vi "demo_ee2.vi"() -> ()   [LabVIEW 2018]
doc: "演示设置基本TCP连接、建立连接后发送数据至指定端口并在完成发送后中止连接的方法。VI设计为TCP连接断开时停止。本范例中发送的数据为随机数数组。"
uses:
  <vilib>/addons/control/pid/NI_PID_autopid.lvlib
panel:
  out "力初始位移":dbl
  out "前馈输出":dbl
  in  "Lower Cut-Off 2":dbl=5.0 caption="截止频率2"
  in  "Lower Cut-Off 1":dbl=5.0 caption="截止频率1"
  out "PID输出":dbl
  in  "重力补偿":dbl=1.15
  in  "力控制频率":dbl=100.0
  in  "位移模块":path caption="文件名"
  in  "力模块":path caption="文件名"
  in  "stop (F) 2":bool caption="停止力控"
  out "力控模块\n气压-位移-力":dynamicdata(graph)
  in  "PID gains":T1={"proportional gain (Kc)"=0.25, "integral time (Ti, min)"=0.05, "derivative time (Td, min)"=0.0} caption="PID增益" {"derivative time (Td, min)" format="%.3f"; "integral time (Ti, min)" format="%.3f"; "proportional gain (Kc)" format="%.3f"}
  in  "output range":cluster{"output high":dbl, "output low":dbl}={"output high"=0.2, "output low"=-0.2} caption="输出范围" {"output low" format="%.2f"; "output high" format="%.2f"}
  in  "a 斜率":dbl=-0.33869
  in  "b 截距":dbl=10.683
  in  "设定力Fd/N":dbl=10.0
  out "力 /N":dynamicdata(graph)
  out "力控模块指令":string
  out "力初始气压":dbl
  in  "stop (F)":bool caption="停止\n位控"
  out "位移模块\n气压-位移-力":dynamicdata(graph)
  in  "位置控制频率":dbl=100.0
  in  "移动速率 mm/s":dbl=0.5
  in  "Flag":i8=2
  out "1/u":dbl(graph)
  in  "力阈值F0/N":dbl=2.0
  out "位置初始气压":dbl
  in  "停止气压":dbl(slide)=4.5 scale=2.5..5.0
  in  "停止 2":bool
  in  "初始气压 /bar":dbl=4.5
  in  "停止":bool
  out "位置模块指令":string
  # "FLag: 1 上升\n        2 下降"
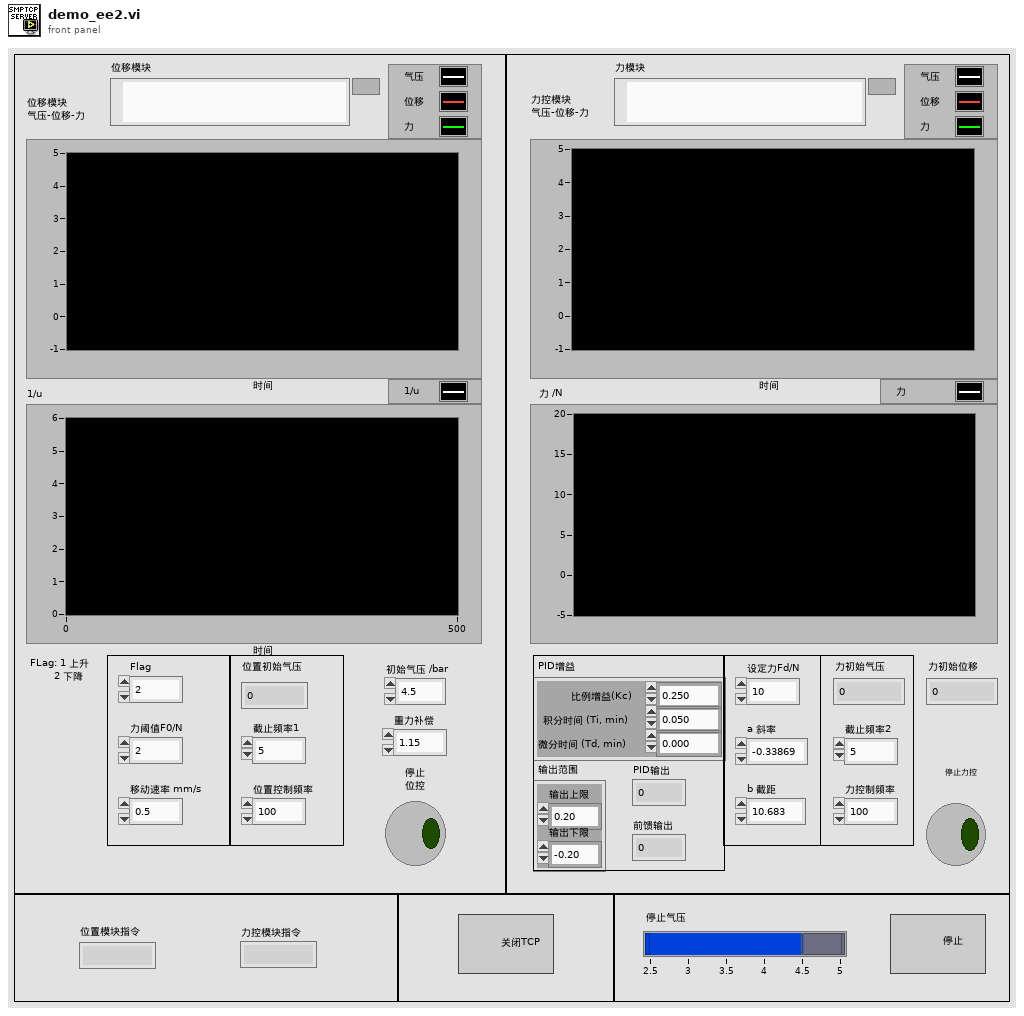
[diagram p1: front panel]
types:
  T1 = cluster{"proportional gain (Kc)":dbl, "integral time (Ti, min)":dbl, "derivative time (Td, min)":dbl}
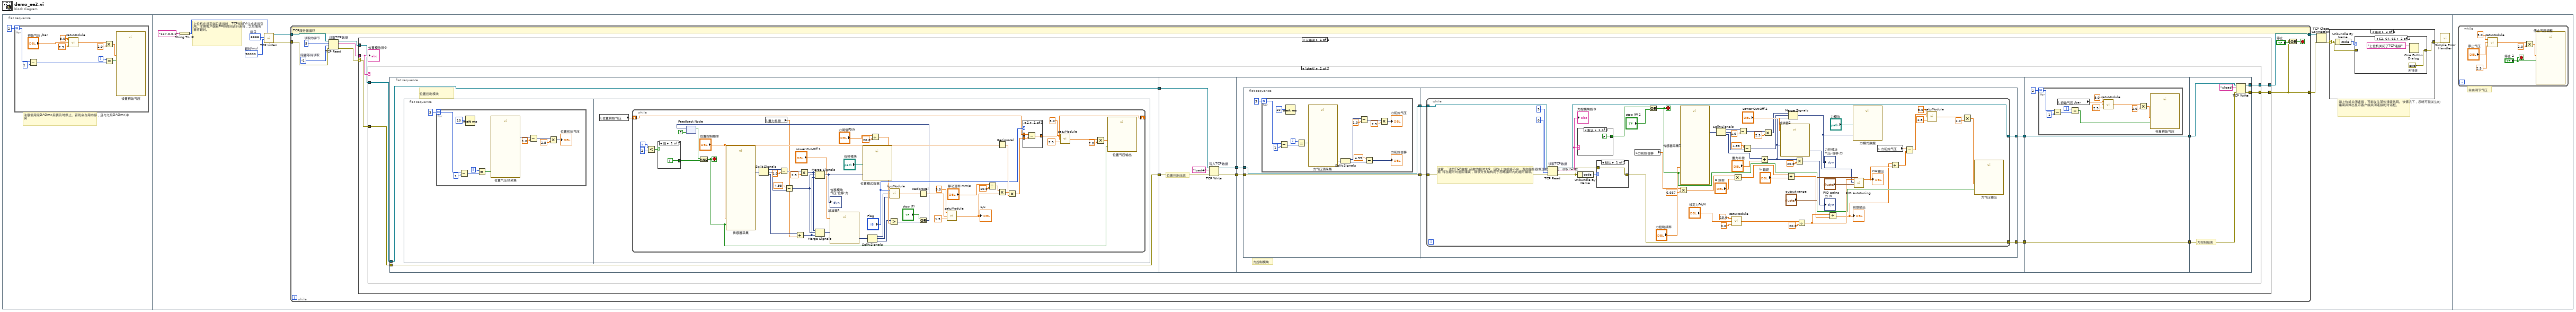
[diagram p0: block diagram]
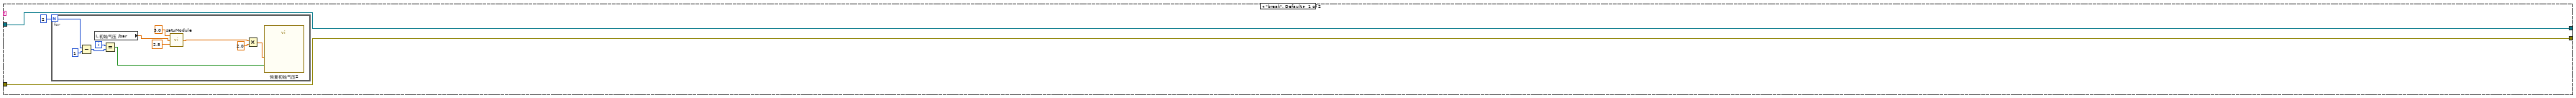
[diagram p4: hidden frame]
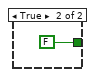
[diagram p5: hidden frame]
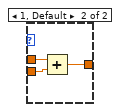
[diagram p6: hidden frame]
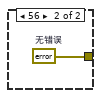
[diagram p7: hidden frame]
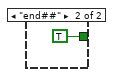
[diagram p8: hidden frame]
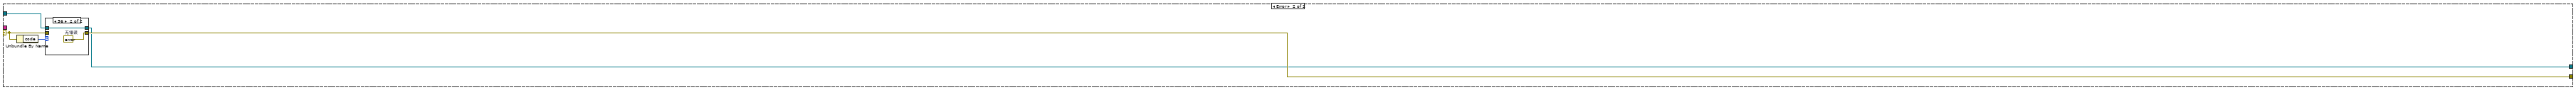
[diagram p9: hidden frame]
diagram:
  n1 = flat-sequence {
    frame #0 {
      # "注意使用完DAQmx后要及时停止。否则会占用内存，且与之后DAQmx冲突"
      n2 = for {
        N: 2 -> [w4]
        i -> [w6]
        n3 = Subtract(x=w4, y=1) -> (x-y=w2:i32)
        n4 = call "satuModule.vi"("min"=2.5, "input"="初始气压 /bar", "max"=5.0) -> ("output"=w11:dbl)
        n5 = Multiply(x=w11, y=2.0 ("x")) -> (x*y=w12:dbl)
        n6 = Equal?(x=w6, y=w2) -> (x = y?=w5:bool)
        n7 = call "设置初始气压"("data"=w12, "stop (T)"=w5) -> ()  [unwired: 16 in, 2 out]
      }
    }
    frame #1 {
      w19 = u16 6666  # 端口
      w20 = 90000  # 超时(ms)
      # "如上位机关闭连接，可能发生某些错误代码。该情况下，忽略可能发生的错误并弹出显示客户端关闭连接的对话框。"
      # "上位机在指定端口连接时，TCP侦听VI生成连接引用。注意客户端有90秒时间进行连接，之后服务器将超时。"
      n8 = String To IP(1:"127.0.0.1") -> (0:w18:u32)
      n9 = call <vilib>:"TCP Listen.vi"("net address"=w18, "timeout ms (wait forever: -1)"=w20, "port"=w19) -> ("error out"=w21:errorcluster, "connection ID"=w22:refnum<k5>)  [unwired: 4 in, 3 out]
      n10 = while {
        tunnel: [w38] -> w13
        tunnel: w22 -> [w37]
        tunnel: w21 -> [w36]
        tunnel: [w32] -> w14
        stop <- w40 stop-if-true
        w30 = -1  # 阻塞等待读取
        w35 = 5  # 读取的字节
        # "TCP服务器循环"
        n11 = TCP Read "读取TCP数据"(connection ID=w37, bytes to read=w35, error in (no error)=w36, 9:w30) -> (connection ID out=w33:refnum<k5>, data out=w31:string, error out=w34:errorcluster)  [unwired: 1 in]
        n12 = case shown="无错误" w34 {
          selector: w34 -> [w43 w263]
          tunnel: [w42 w262] -> w38
          tunnel: w33 -> [w44 w261]
          tunnel: [w41 w260] -> w32
          tunnel: w31 -> [w45 _]
          frame No Error {
            n13 = case shown="\"start\"" w45 {
              tunnel: w44 -> [w47 w64]
              tunnel: w43 -> [w48 w71]
              tunnel: [w48 w69] -> w42
              tunnel: [w47 w66] -> w41
              frame "break", Default {
                n14 = for {
                  N: 2 -> [w53]
                  i -> [w50]
                  n15 = Subtract(x=w53, y=1) -> (x-y=w51:i32)
                  n16 = local read "初始气压 /bar"() -> (w54:dbl)
                  n17 = Equal?(x=w50, y=w51) -> (x = y?=w49:bool)
                  n18 = call "satuModule.vi"("min"=2.5, "input"=w54, "max"=5.0) -> ("output"=w58:dbl)
                  n19 = Multiply(x=w58, y=2.0 ("x")) -> (x*y=w59:dbl)
                  n20 = call "恢复初始气压2"("data"=w59, "stop (T)"=w49) -> ()  [unwired: 16 in, 2 out]
                }
              }
              frame "start" {
                n21 = flat-sequence {
                  tunnel: w71 -> [w73]
                  tunnel: [w73] -> w70
                  tunnel: [w72] -> w65
                  tunnel: w64 -> [w72]
                  tunnel: w70 -> [w151]
                  tunnel: [w150] -> w68
                  tunnel: [w149] -> w67
                  tunnel: w65 -> [w148]
                  tunnel: w68 -> [w155]
                  tunnel: w67 -> [w157]
                  tunnel: [w154] -> w62
                  tunnel: [w153] -> w60
                  tunnel: [w243] -> w63
                  tunnel: w62 -> [w243]
                  tunnel: [w242] -> w61
                  tunnel: w60 -> [w242]
                  tunnel: [w258] -> w66
                  tunnel: [w257] -> w69
                  tunnel: w63 -> [w256]
                  tunnel: w61 -> [w255]
                  frame #0 {
                    # "位置控制模块"
                    n22 = flat-sequence {
                      frame #0 {
                        n23 = for {
                          N: 3 -> [w77]
                          i -> [w80]
                          n24 = Subtract(x=w77, y=1) -> (x-y=w75:i32)
                          n25 = Wait (ms)(milliseconds to wait=u32 10 ("等待时间（毫秒）")) -> ()  [unwired: 1 out]
                          n26 = Equal?(x=w80, y=w75) -> (x = y?=w79:bool)
                          n27 = call "位置气压预采集"("stop (T)"=w79) -> ("data"=w82:dynamicdata)  [unwired: 16 in, 2 out]
                          n28 = Subtract(x=w82, y=1.0) -> (x-y=w85:dynamicdata)
                          n29 = Multiply(x=w85, y=2.5) -> (x*y=→"位置初始气压":dynamicdata)
                        }
                      }
                      frame #1 {
                        n30 = local read "位置初始气压"() -> (w86:dbl)
                        n31 = while {
                          shift-right: [w113] -> _
                          shift-left: w86 -> [w112]
                          i -> [w100]
                          stop <- w101 stop-if-true
                          n32 = Less?(x=w100, y=2) -> (x < y?=w98:bool)
                          n33 = case shown="假" w98 {
                            tunnel: [TRUE FALSE] -> w97
                            frame False {
                            }
                            frame True {
                            }
                          }
                          n34 = feedback #1(FALSE) -> (w102:bool)
                          n35 = And(x=w102, y=w97) -> (x .and. y?=w101:bool)
                          n36 = call "传感器采集"("速率"="位置控制频率", "stop (F)"=w101) -> ("data"=w136:dynamicdata)  [unwired: 14 in, 3 out]
                          n37 = Split Signals(w136) -> (w135:dynamicdata, w133:dynamicdata, w130:dynamicdata)  [unwired: 3 in]
                          n38 = local read "重力补偿"() -> (w96:dbl)
                          n39 = Subtract(x=w135, y=1.0) -> (x-y=w138:dynamicdata)
                          n40 = Subtract(x=4.95, y=w133) -> (x-y=w94:dynamicdata)
                          n41 = Add(x=w130, y=w96) -> (x+y=w93:dynamicdata)
                          n42 = Multiply(x=w138, y=2.5) -> (x*y=w95:dynamicdata)
                          n43 = Merge Signals(w95, w94, w93) -> (w107:dynamicdata)
                          "位移模块\n气压-位移-力" <- w107
                          n44 = Merge Signals(w95, w94, w93) -> (w92:dynamicdata)
                          n45 = call "滤波器1"("Lower Cut-Off"="Lower Cut-Off 1", "Signal"=w92) -> ("Filtered Signal"=w87:dynamicdata)  [unwired: 8 in, 1 out]
                          n46 = call "位置模式数据"("Signals"=w107, "Filename"="位移模块") -> ()  [unwired: 15 in, 3 out]
                          n47 = Split Signals(w87) -> (w91:dynamicdata, w90:dynamicdata, w89:dynamicdata)  [unwired: 3 in]
                          n48 = Divide(x="力阈值F0/N", y=20.0) -> (x/y=w109:dbl)
                          n49 = Greater?(x=w89, y=w109) -> (0:w105:dynamicdata)
                          n50 = call "hysModule.vi"("cur_x"=w90, "cur_p"=w91, "flag"="Flag") -> ("u"=w116:dbl)
                          n51 = Reciprocal(x=w116) -> (1/x=w115:dbl)
                          n52 = Or(x="stop (F)", y=w105) -> (x .or. y?=w104:dynamicdata)
                          n53 = feedback-in #1(w104) -> ()
                          n54 = call "satuModule.vi"("min"=1.5, "input"=w115, "max"=5.0) -> ("output"=w114:dbl)
                          "1/u" <- w114
                          n55 = Divide(x="移动速率 mm/s", y=10.0) -> (x/y=w124:dbl)
                          n56 = Reciprocal(x="位置控制频率") -> (1/x=w121:dbl)
                          n57 = Multiply(x=w124, y=w114) -> (x*y=w122:dbl)
                          n58 = Multiply(x=w122, y=w121) -> (x*y=w119:dbl)
                          n59 = case shown="2" "Flag" {
                            tunnel: [w144 w147] -> w113
                            tunnel: w119 -> [w143 w146]
                            tunnel: w112 -> [w142 w145]
                            frame 2 {
                              n60 = Subtract(x=w142, y=w143) -> (x-y=w144:dbl)
                            }
                            frame 1, Default {
                              n61 = Add(x=w145, y=w146) -> (x+y=w147:dbl)
                            }
                          }
                          n62 = call "satuModule.vi"("min"=2.5, "input"=w113, "max"=5.0) -> ("output"=w127:dbl)
                          n63 = Multiply(x=w127, y=2.0 ("x")) -> (x*y=w132:dbl)
                          n64 = call "位置气压输出"("data"=w132, "stop (T)"=w101) -> ()  [unwired: 16 in, 2 out]
                        }
                      }
                    }
                  }
                  frame #1 {
                    # "位置控制结束"
                    n65 = TCP Write "写入TCP数据"(connection ID=w148, data in="load#" ("数据输入"), error in (no error)=w151) -> (connection ID out=w149:refnum<k5>, error out=w150:errorcluster)  [unwired: 2 out]
                  }
                  frame #2 {
                    # "力控制模块"
                    n66 = flat-sequence {
                      tunnel: [w161] -> w158
                      tunnel: w157 -> [w161]
                      tunnel: [w160] -> w156
                      tunnel: w155 -> [w160]
                      tunnel: w158 -> [w180]
                      tunnel: w156 -> [w179]
                      tunnel: [w178] -> w154
                      tunnel: [w177] -> w153
                      frame #0 {
                        n67 = for {
                          N: 3 -> [w169]
                          i -> [w172]
                          n68 = Subtract(x=w169, y=1) -> (x-y=w168:i32)
                          n69 = Wait (ms)(milliseconds to wait=u32 10 ("等待时间（毫秒）")) -> ()  [unwired: 1 out]
                          n70 = Equal?(x=w172, y=w168) -> (x = y?=w171:bool)
                          n71 = call "力气压预采集"("stop (T)"=w171) -> ("data"=w166:dynamicdata)  [unwired: 16 in, 2 out]
                          n72 = Split Signals(w166) -> (w165:dynamicdata, w164:dynamicdata)  [unwired: 2 in]
                          n73 = Subtract(x=w165, y=1.0) -> (x-y=w176:dynamicdata)
                          n74 = Subtract(x=4.95, y=w164) -> (x-y=→"力初始位移":dynamicdata)
                          n75 = Multiply(x=w176, y=2.5) -> (x*y=→"力初始气压":dynamicdata)
                        }
                      }
                      frame #1 {
                        n76 = while {
                          tunnel: w180 -> [w199]
                          tunnel: w179 -> [w198]
                          tunnel: [w197] -> w178
                          tunnel: [w196] -> w177
                          stop <- w192 stop-if-true
                          # "注意，“读取TCP数据”函数的超时为0，因为上位机将不会一直向服务器发送数据。由于“读取TCP数据”将在超时时返回错误，错误分支结构用于忽略循环内的超时错误。"
                          n77 = TCP Read "读取TCP数据"(connection ID=w199, bytes to read=5 ("读取的字节"), error in (no error)=w198, 9:0 ("超时毫秒(25000)")) -> (connection ID out=w197:refnum<k5>, data out=w204:string, error out=w200:errorcluster)  [unwired: 1 in]
                          "力控模块指令" <- w204
                          n78 = case shown="默认" w204 {
                            tunnel: [FALSE TRUE] -> w202
                            frame Default {
                            }
                            frame "end##" {
                            }
                          }
                          n79 = Unbundle By Name(w200) -> ("code"=w201:i32)
                          n80 = case shown="默认" w201 {
                            tunnel: w200 -> [w237 _]
                            tunnel: [w237 w238] -> w196
                            frame Default {
                            }
                            frame 56 {
                              w238 = errorcluster {"status"=FALSE, "code"=0, "source"=""}  # 无错误
                            }
                          }
                          n81 = local read "力初始位移"() -> (w182:dbl)
                          n82 = Or(x=w202, y="stop (F) 2") -> (x .or. y?=w192:bool)
                          n83 = Multiply(x=w182, y=6.667) -> (x*y=w227:dbl)
                          n84 = call "传感器采集2"("速率"="力控制频率", "stop (F)"=w192) -> ("data"=w233:dynamicdata)  [unwired: 14 in, 3 out]
                          n85 = Split Signals(w233) -> (w223:dynamicdata, w221:dynamicdata, w220:dynamicdata)  [unwired: 3 in]
                          n86 = call "satuModule.vi"("min"=0.0 ("下限"), "input"="设定力Fd/N", "max"=15.0) -> ("output"=w213:dbl)
                          n87 = Multiply(x=w227, y="a 斜率") -> (x*y=w224:dbl)
                          n88 = Subtract(x=w223, y=1.0) -> (x-y=w235:dynamicdata)
                          n89 = Subtract(x=4.95, y=w221) -> (x-y=w186:dynamicdata)
                          n90 = Add(x=w220, y="重力补偿") -> (x+y=w184:dynamicdata)
                          n91 = Multiply(x=w235, y=2.5) -> (x*y=w187:dynamicdata)
                          n92 = call "滤波器2"("Lower Cut-Off"="Lower Cut-Off 2", "Signal"=w184) -> ("Filtered Signal"=w183:dynamicdata)  [unwired: 8 in, 1 out]
                          n93 = Add(x=w224, y="b 截距") -> (x+y=w181:dbl)
                          n94 = Merge Signals(w187, w186, w184) -> (w195:dynamicdata)
                          "力控模块\n气压-位移-力" <- w195
                          n95 = Multiply(x=w184, y=20.0) -> (x*y=→"力 /N":dynamicdata)
                          n96 = Divide(x=w213, y=20.0) -> (x/y=w211:dbl)
                          n97 = Divide(x=w211, y=w181) -> (x/y=w185:dbl)
                          "前馈输出" <- w185
                          n98 = call "力模式数据"("Signals"=w195, "Filename"="力模块") -> ()  [unwired: 15 in, 3 out]
                          n99 = call <vilib>:"PID Autotuning.vi"("output range"="output range", "PID gains"="PID gains", "process variable"=w183, "setpoint"=w211) -> ("output"=w189:dbl)  [unwired: 4 in, 3 out]
                          "PID输出" <- w189
                          n100 = local read "力初始气压"() -> (w207:dbl)
                          n101 = Add(x=w185, y=w189) -> (x+y=w219:dbl)
                          n102 = Subtract(x=w207, y=w219) -> (x-y=w218:dbl)
                          n103 = call "satuModule.vi"("min"=2.5 ("下限"), "input"=w218, "max"=5.0) -> ("output"=w216:dbl)
                          n104 = Multiply(x=w216, y=2.0) -> (x*y=w228:dbl)
                          n105 = call "力气压输出"("data"=w228, "stop (T)"=w192) -> ()  [unwired: 16 in, 2 out]
                        }
                      }
                    }
                  }
                  frame #3 {
                    n106 = for {
                      N: 2 -> [w246]
                      i -> [w248]
                      n107 = Subtract(x=w246, y=1) -> (x-y=w244:i32)
                      n108 = local read "初始气压 /bar"() -> (w250:dbl)
                      n109 = Equal?(x=w248, y=w244) -> (x = y?=w247:bool)
                      n110 = call "satuModule.vi"("min"=2.5, "input"=w250, "max"=5.0) -> ("output"=w253:dbl)
                      n111 = Multiply(x=w253, y=2.0 ("x")) -> (x*y=w254:dbl)
                      n112 = call "恢复初始气压"("data"=w254, "stop (T)"=w247) -> ()  [unwired: 16 in, 2 out]
                    }
                  }
                  frame #4 {
                    # "力控制结束"
                    n113 = TCP Write(connection ID=w256, data in="uload" ("数据输入"), error in (no error)=w255) -> (connection ID out=w258:refnum<k5>, error out=w257:errorcluster)  [unwired: 2 out]
                  }
                }
              }
            }
            "位置模块指令" <- w45
          }
          frame Error {
            n114 = Unbundle By Name(w263) -> ("code"=w264:i32)
            n115 = case shown="56" w264 {
              tunnel: w263 -> [w266 _]
              tunnel: [w266 w268] -> w262
              tunnel: w261 -> [w265 w267]
              tunnel: [w265 w267] -> w260
              frame Default {
              }
              frame 56 {
                w268 = errorcluster {"status"=FALSE, "code"=0, "source"=""}  # 无错误
              }
            }
          }
        }
        n116 = Compound Arithmetic op=OR ("复合运算")(w38, "停止") -> (w40:bool)
      }
      n117 = TCP Close Connection ("关闭TCP连接")(connection ID=w14, error in (no error)=w13) -> (error out=w15:errorcluster)  [unwired: 2 out]
      n118 = case shown="错误" w15 {
        selector: w15 -> [w23 w25]
        tunnel: [w23 w24] -> w16
        frame No Error {
        }
        frame Error {
          n119 = Unbundle By Name(w25) -> ("code"=w26:i32)
          n120 = case shown="62, 64, 66" w26 {
            tunnel: w25 -> [w27 _]
            tunnel: [w27 w29] -> w24
            frame Default {
            }
            frame 62, 64, 66 {
              w29 = errorcluster {"status"=FALSE, "code"=0, "source"=""}  # 无错误
              n121 = One Button Dialog(message="上位机关闭了TCP连接" ("消息")) -> ()  [unwired: 1 in, 1 out]
            }
          }
        }
      }
      n122 = call <vilib>:"Simple Error Handler.vi"("error in (no error)"=w16) -> ()  [unwired: 1 in, 8 out]
    }
    frame #2 {
      # "自由调节气压"
      n123 = while {
        stop <- "停止 2" stop-if-true
        n124 = call "satuModule.vi"("min"=2.5, "input"="停止气压", "max"=5.0) -> ("output"=w274:dbl)
        n125 = Multiply(x=w274, y=2.0 ("x")) -> (x*y=w275:dbl)
        n126 = call "停止气压调整"("data"=w275, "stop (T)"="停止 2") -> ()  [unwired: 16 in, 2 out]
      }
    }
  }
